vi "Arcade arm.vi"() -> ()   [LabVIEW 2014]
uses:
  <vilib>/Utility/inputDevices.llb/joystickAcquire.vi
panel:
  out "Image":T1(plugin-control)
  out "hand angle":dbl(knob) scale=180.0..-180.0
  in  "hand length":dbl
  in  "y":dbl
  in  "x":dbl
  out "arm angle":dbl(knob) scale=180.0..-180.0
  out "arm length":dbl(slide) scale=0.0..1000.0
  in  "hand angle relative to ground":dbl
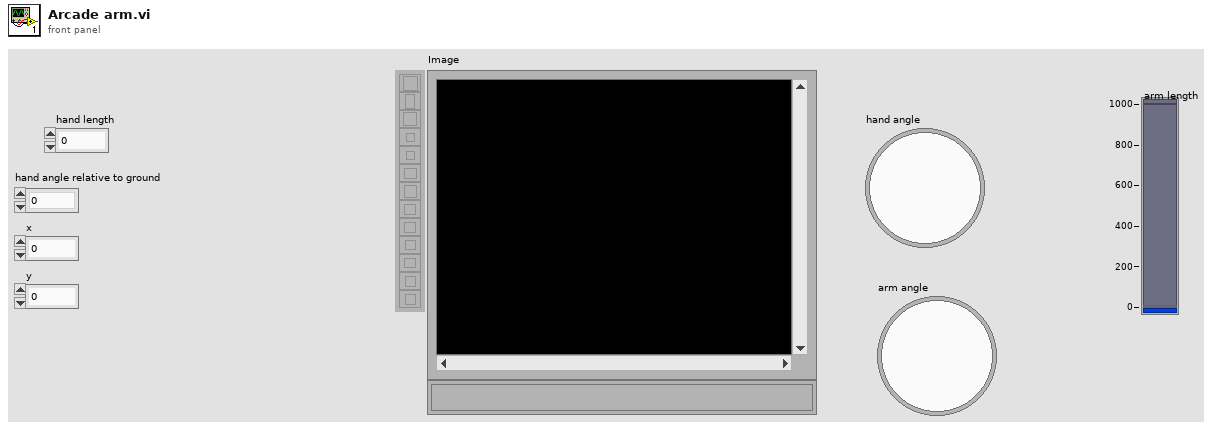
[diagram p1: front panel]
types:
  T1 = typedef "IMAQ Image.ctl" = refnum<image>
  T2 = cluster{"Left":i32, "Top":i32, "Right":i32, "Bottom":i32}
  T3 = cluster{"X axis":i32, "Y axis":i32, "Z axis":i32, "X axis rotation":i32, "Y axis rotation":i32, "Z axis rotation":i32, "U axis":i32, "V axis":i32}
  T4 = cluster{"X axis":dbl, "Y axis":dbl, "Z axis":dbl, "X axis rotation":dbl, "Y axis rotation":dbl, "Z axis rotation":dbl, "U axis":dbl, "V axis":dbl}
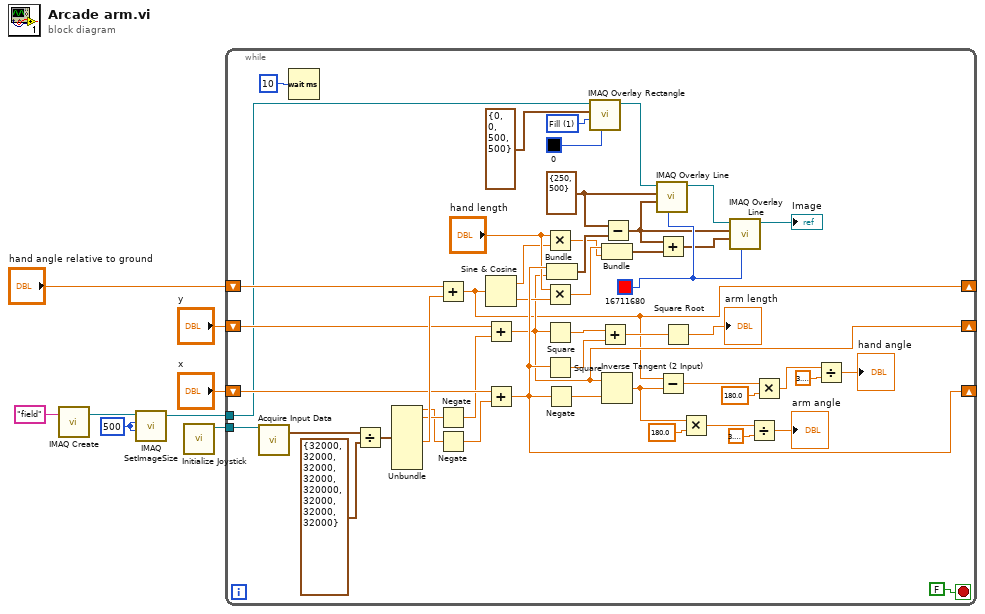
[diagram p0: block diagram]
diagram:
  w2 = 500 ("X Resolution")
  n1 = call "IMAQ Create"("Image Name"="field") -> ("New Image"=w3:T1)  [unwired: 4 in, 1 out]
  n2 = call "IMAQ SetImageSize"("Y Resolution"=w2, "X Resolution"=w2, "Image"=w3) -> ("Image Out"=w1:T1)  [unwired: 2 in, 1 out]
  n3 = call <vilib>:"Initialize Joystick.vi"() -> ("device ID"=w8:refnum<k1>)  [unwired: 10 in, 1 out]
  n4 = while {
    tunnel: w8 -> [w49]
    shift-right: [w12] -> _
    shift-left: "hand angle relative to ground" -> [w47]
    shift-right: [w13] -> _
    shift-left: "y" -> [w43]
    shift-right: [w30] -> _
    shift-left: "x" -> [w41]
    tunnel: w1 -> [w35]
    stop <- FALSE stop-if-true
    w26 = u32 16711680 ("Color")
    w27 = cluster{"X":i32, "Y":i32} {"X"=250, "Y"=500} ("Start Point")
    w32 = u32 1 items=["Frame", "Fill", "Highlight"] ("Drawing Mode (Frame)")
    n5 = call-poly <vilib>:"Acquire Input Data.vi"("device ID"=w49) -> ("axis info"=w48:T3)  [unwired: 14 in, 4 out]
    n6 = Wait (ms)(milliseconds to wait=u32 10) -> ()  [unwired: 1 out]
    n7 = Divide(x=w48, y=T3 {"X axis"=32000, "Y axis"=32000, "Z axis"=32000, "X axis rotation"=32000, "Y axis rotation"=320000, "Z axis rotation"=32000, "U axis"=32000, "V axis"=32000}) -> (x/y=w46:T4)
    n8 = Unbundle(w46) -> ("X axis"=w40:dbl, "Y axis"=w42:dbl, "Y axis rotation"=w44:dbl)  [unwired: 5 out]
    n9 = Add(x=w47, y=w44) -> (x+y=w12:dbl)
    n10 = Negate(x=w42) -> (-x=w15:dbl)
    n11 = Negate(x=w40) -> (-x=w14:dbl)
    n12 = Sine & Cosine(0:w12) -> (1:w18:dbl, 2:w19:dbl)
    n13 = Add(x=w43, y=w15) -> (x+y=w13:dbl)
    n14 = Add(x=w41, y=w14) -> (x+y=w30:dbl)
    n15 = Multiply(x="hand length", y=w18) -> (x*y=w21:dbl)
    n16 = Multiply(x="hand length", y=w19) -> (x*y=w22:dbl)
    n17 = Square(x=w13) -> (x^2=w56:dbl)
    n18 = Square(x=w30) -> (x^2=w55:dbl)
    n19 = Negate(x=w30) -> (-x=w11:dbl)
    n20 = Bundle(w30, w13) -> (w29:cluster{dbl, dbl})  [unwired: 1 in]
    n21 = call "IMAQ Overlay Rectangle"("Color"=u32 0, "Drawing Mode (Frame)"=w32, "Rectangle"=T2 {"Left"=0, "Top"=0, "Right"=500, "Bottom"=500}, "Image"=w35) -> ("Image Out"=w31:T1)  [unwired: 6 in, 1 out]
    n22 = Add(x=w56, y=w55) -> (x+y=w57:dbl)
    n23 = Bundle(w22, w21) -> (w23:cluster{dbl, dbl})  [unwired: 1 in]
    n24 = Inverse Tangent (2 Input)(1:w11, 2:w13) -> (0:w39:dbl)
    n25 = Subtract(x=w27, y=w29) -> (x-y=w25:cluster{dbl, dbl})
    n26 = call "IMAQ Overlay Line"("Color"=w26, "End Point"=w25, "Start Point"=w27, "Image"=w31) -> ("Image Out"=w28:T1)  [unwired: 6 in, 1 out]
    n27 = Add(x=w25, y=w23) -> (x+y=w24:cluster{dbl, dbl})
    n28 = Subtract(x=w12, y=w39) -> (x-y=w17:dbl)
    n29 = Square Root(x=w57) -> (sqrt(x)=→"arm length":dbl)
    n30 = Multiply(x=w39, y=180.0) -> (x*y=w54:dbl)
    n31 = call "IMAQ Overlay Line"("Color"=w26, "End Point"=w24, "Start Point"=w25, "Image"=w28) -> ("Image Out"=→"Image":T1)  [unwired: 6 in, 1 out]
    n32 = Divide(x=w54, y=3.141592653589793) -> (x/y=→"arm angle":dbl)
    n33 = Multiply(x=w17, y=180.0) -> (x*y=w53:dbl)
    n34 = Divide(x=w53, y=3.141592653589793) -> (x/y=→"hand angle":dbl)
  }
